vi "UpdateLayerData.vi"(4 "Type":T1, 6 "Overwrite?":bool, 8 "error in":errorcluster, 9 "LayerName":string, 10 "new picture":picture, 11 "Active Layer":refnum<class "Layer.lvclass">) -> (0 "error out":errorcluster, 3 "Layer.lvclass out":refnum<class "Layer.lvclass">)   [LabVIEW 2021, in "Layer.lvclass"]
doc: "If the flag Overwrite is true, the incoming Glyph is merged with the already existing User Layer data. \nThe new Layer Name is only applied if the Active User Layer is not called 'NI_Library\"."
uses:
  Layer.lvclass
  Controls/LayerType.ctl
  lv_icon.lvlib
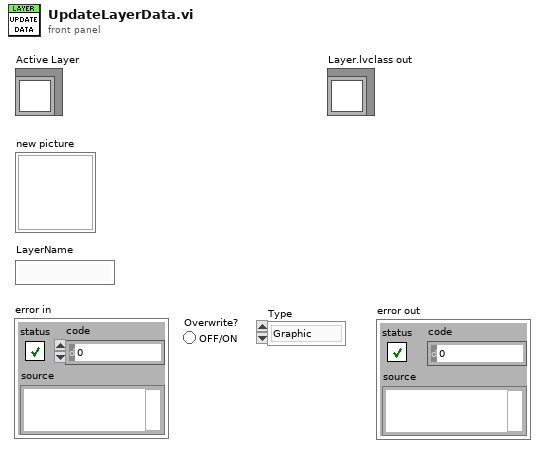
[diagram p1: front panel]
types:
  T1 = typedef "LayerType.ctl" = enum16{"Graphic", "Text", "Tool", "Graphic Drop"}
  T2 = typedef "Layer.ctl" = cluster{"LayerIcon":picture, "LayerName":string, "Opacity":u8, "Visibility?":bool}
  T3 = typedef "LVPoint32TypeDef.ctl" = cluster{"Horizontal":i32, "Vertical":i32}
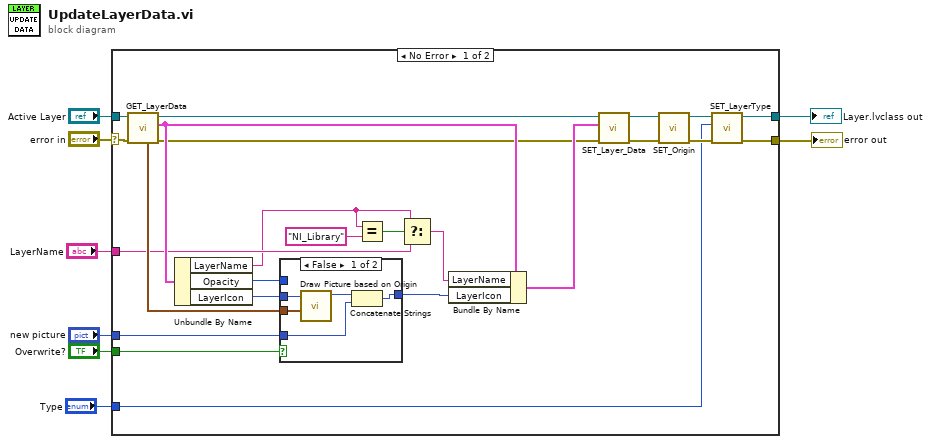
[diagram p0: block diagram]
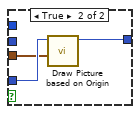
[diagram p2: hidden frame]
diagram:
  n1 = case shown="No Error" "error in" {
    selector: "error in" -> [w24 w41]
    tunnel: "new picture" -> [w15 _]
    tunnel: [w17 w41] -> w7
    tunnel: [w18 w42] -> w6
    tunnel: "Active Layer" -> [w25 w42]
    tunnel: "Overwrite?" -> [w23 _]
    tunnel: "LayerName" -> [w13 _]
    tunnel: "Type" -> [w16 _]
    frame No Error {
      n2 = call-dynamic "GET_LayerData.vi"("error in (no error)"=w24, "Layer.lvclass in"=w25) -> ("error out"=w9:errorcluster, "Data"=w29:T2, "Layer.lvclass out"=w31:refnum<class "Layer.lvclass">, "Origin"=w27:T3)  [unwired: 6 out]
      n3 = Unbundle By Name(w29) -> ("LayerName"=w12:string, "Opacity"=w28:u8, "LayerIcon"=w26:picture)
      n4 = case shown="False" w23 {
        tunnel: [w33 w39] -> w30
        tunnel: w28 -> [_ _]
        tunnel: w27 -> [w37 w38]
        tunnel: w26 -> [w36 _]
        tunnel: w15 -> [w34 w40]
        frame False {
          n5 = call "Draw Picture based on Origin.vi"("Origin"=w37, "LayerIcon in"=w36) -> ("LayerIcon out"=w35:picture)  [unwired: 1 in, 8 out]
          n6 = Concatenate Strings(w35, w34) -> (w33:picture)
        }
        frame True {
          n7 = call "Draw Picture based on Origin.vi"("Origin"=w38, "LayerIcon in"=w40) -> ("LayerIcon out"=w39:picture)  [unwired: 1 in, 8 out]
        }
      }
      n8 = Equal?(x=w12, y="NI_Library") -> (x = y?=w10:bool)
      n9 = Select(t=w12, s=w10, f=w13) -> (s? t:f=w14:string)
      n10 = Bundle By Name(cluster=w29, "LayerName"=w14, "LayerIcon"=w30) -> (w32:T2)
      n11 = call-dynamic "SET_Layer_Data.vi"("error in (no error)"=w9, "Data"=w32, "Layer.lvclass in"=w31) -> ("error out"=w22:errorcluster, "Layer.lvclass out"=w21:refnum<class "Layer.lvclass">)  [unwired: 1 in, 6 out]
      n12 = call-dynamic "SET_Origin.vi"("error in (no error)"=w22, "Layer.lvclass in"=w21) -> ("error out"=w20:errorcluster, "Layer.lvclass out"=w19:refnum<class "Layer.lvclass">)  [unwired: 1 in, 7 out]
      n13 = call-dynamic "SET_LayerType.vi"("error in (no error)"=w20, "Type"=w16, "Layer.lvclass in"=w19) -> ("error out"=w17:errorcluster, "Layer.lvclass out"=w18:refnum<class "Layer.lvclass">)  [unwired: 7 out]
    }
    frame Error {
    }
  }
  "error out" <- w7
  "Layer.lvclass out" <- w6
